vi "ParseResponseCode.vi"(11 "Response Header":string) -> (3 "response code (200)":T1=200 items=["100"=100, "101"=101, "200"=200, "201"=201, "202"=202, "203"=203, "204"=204, "205"=205, "206"=206, "300"=300, "301"=301, "302"=302, "303"=303, "304"=304, "305"=305, "306"=306, "307"=307, "400"=400, "401"=401, "402"=402, "403"=403, "404"=404, "405"=405, "406"=406, "407"=407, "408"=408, "409"=409, "410"=410, "411"=411, "412"=412, "413"=413, "414"=414, "415"=415, "416"=416, "417"=417, "500"=500, "501"=501, "502"=502, "503"=503, "504"=504, "505"=505])   [LabVIEW 2020, in "StashRoyale.lvclass"]
uses:
  StashRoyale.lvclass
  ctl_ErrorCodes.ctl
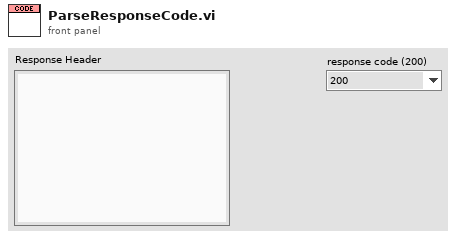
[diagram p1: front panel]
types:
  T1 = typedef "StashRoyale.lvclass/ctl_ErrorCodes.ctl" = i32
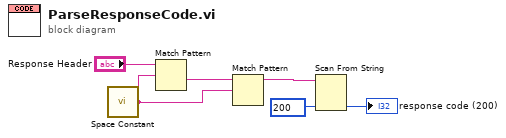
[diagram p0: block diagram]
diagram:
  w2 = T1 200 items=["100"=100, "101"=101, "200"=200, "201"=201, "202"=202, "203"=203, "204"=204, "205"=205, "206"=206, "300"=300, "301"=301, "302"=302, "303"=303, "304"=304, "305"=305, "306"=306, "307"=307, "400"=400, "401"=401, "402"=402, "403"=403, "404"=404, "405"=405, "406"=406, "407"=407, "408"=408, "409"=409, "410"=410, "411"=411, "412"=412, "413"=413, "414"=414, "415"=415, "416"=416, "417"=417, "500"=500, "501"=501, "502"=502, "503"=503, "504"=504, "505"=505] ("response code (200)")
  n1 = call <vilib>:"Space Constant.vi"() -> ("String"=w4:string)
  n2 = Match Pattern(string="Response Header", regular expression=w4) -> (after substring=w5:string)  [unwired: 1 in, 3 out]
  n3 = Match Pattern(string=w5, regular expression=w4) -> (before substring=w3:string)  [unwired: 1 in, 3 out]
  n4 = Scan From String(input string=w3, default 1=w2) -> (output 1=→"response code (200)":T1)  [unwired: 3 in, 3 out]
